vi "RunStimOnRailsThenOnTurns.vi"() -> ()   [LabVIEW 2019]
uses:
  Parameters.ctl
  StimOnRailsThenOnTurns/StimOnRailsThenOnTurnsInputCluster.ctl
  DetectSuppressionDuration/StimOnRailsThenOnTurns.lvclass
  D:/Github_repos/ProjectAPI/LabviewVIs/StimulusObject.lvclass
panel:
  in  "StimOnRailsThenOnTurnsInputCluster":T1={"Constant Intensity (uW/mm^2, negative is blue)"=0.0, "dot radius (mm)"=0.3, "Intensities (uW/mm^2, negative is blue)"=[], "Durations (s)"=[], "Inter trigger interval (s)"=10.0, "Ellipse Ratio Trigger Point"=5.0, "Delays (s)"=[]}
  out "error IO":errorcluster
  in  "SSH password 2":string
  in  "SSH user name 2":string
  in  "Start":bool
  in  "Wait Before Recording (s)":u32
  in  "SSH password":string
  in  "SSH user name":string
  in  "Last Experiment of the Day":bool
  in  "Tags":string
  out "Parameters":T2 {"FW_WormLengthSD" format="%#.6e"}
  # "Faux Worm Drawing"
  # "Tracking"
  # "Temporal Calibration"
  # "Stimulus Generation"
  # "Median Filtering"
  # "Experimental Settings"
  # "Camera and Projector Settings"
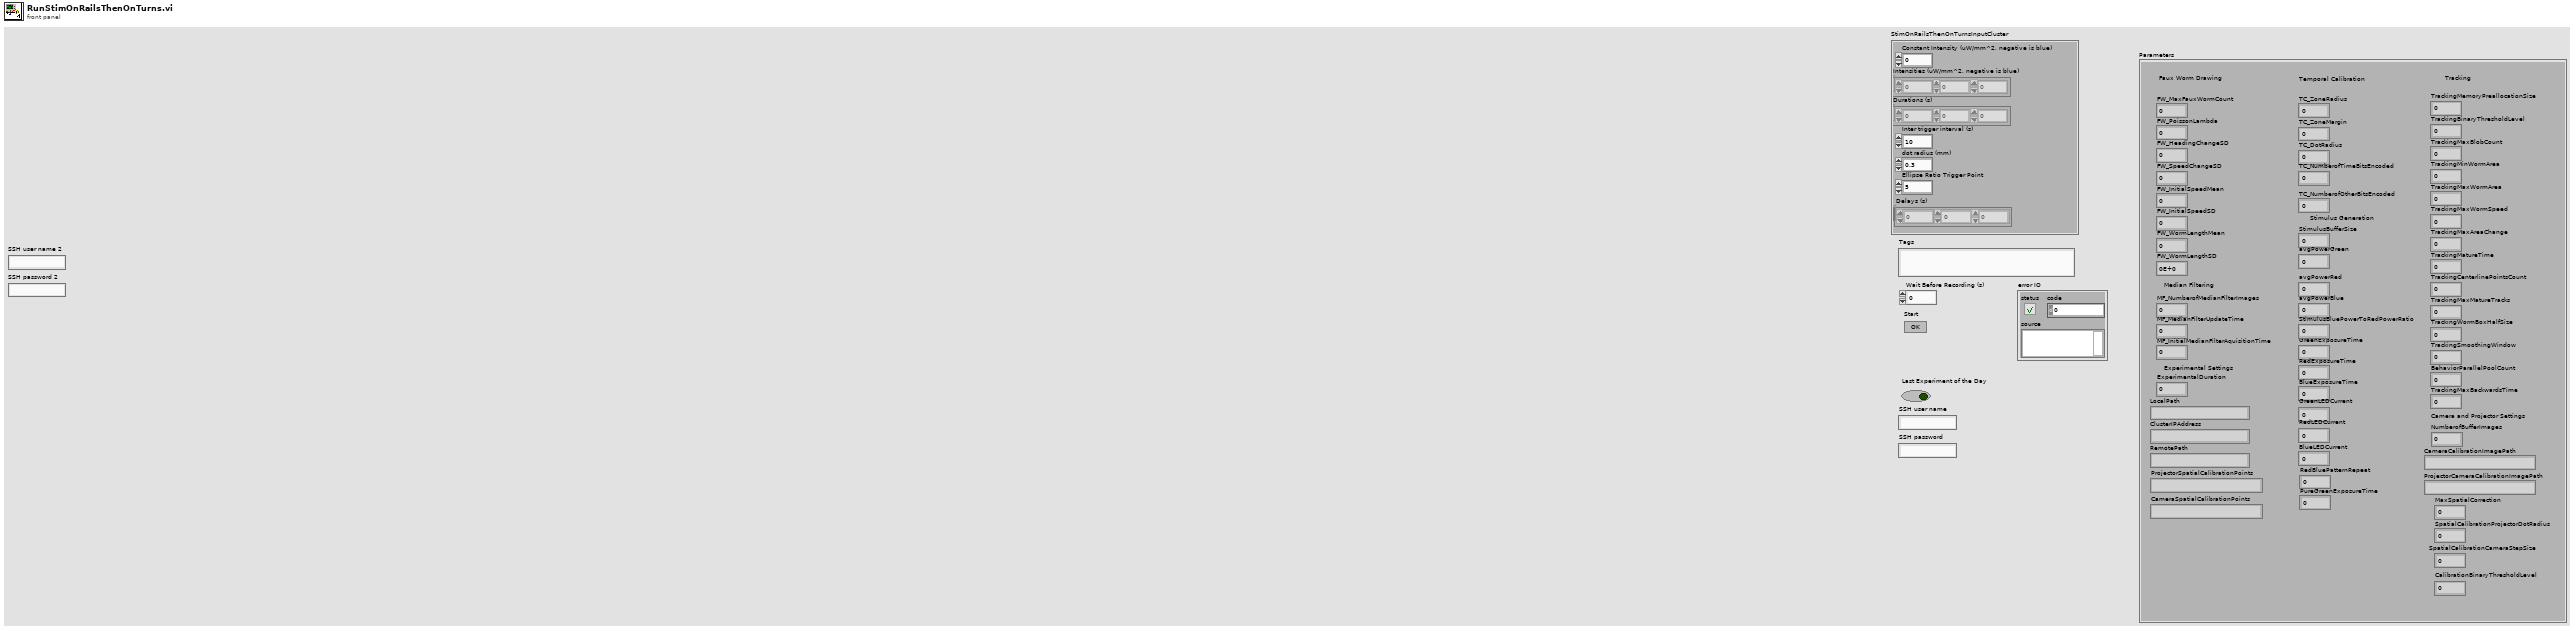
[diagram p1: front panel]
types:
  T1 = typedef "StimOnRailsThenOnTurns.lvclass/StimOnRailsThenOnTurnsInputCluster.ctl" = cluster{"Constant Intensity (uW/mm^2, negative is blue)":sgl, "dot radius (mm)":sgl, "Intensities (uW/mm^2, negative is blue)":sgl[], "Durations (s)":sgl[], "Inter trigger interval (s)":dbl, "Ellipse Ratio Trigger Point":sgl, "Delays (s)":sgl[]}
  T2 = typedef "Parameters.ctl" = cluster{"FW_MaxFauxWormCount":i32, "FW_PoissonLambda":dbl, "FW_HeadingChangeSD":dbl, "FW_SpeedChangeSD":dbl, "FW_InitialSpeedMean":dbl, "FW_InitialSpeedSD":dbl, "FW_WormLengthMean":dbl, "FW_WormLengthSD":dbl, "MF_NumberofMedianFilterImages":i32, "MF_MedianFilterUpdateTime":i32, "MF_InitialMedianFilterAquisitionTime":dbl, "ExperimentalDuration":i32, "TC_ZoneRadius":i32, "TC_ZoneMargin":i32, "TC_DotRadius":dbl, "TC_NumberofTimeBitsEncoded":i32, "TC_NumberofOtherBitsEncoded":i32, "NumberofBufferImages":sgl, "CameraCalibrationImagePath":string, "ProjectorCameraCalibrationImagePath":string, "StimulusBufferSize":i32, "TrackingMemoryPreallocationSize":i32, "TrackingBinaryThresholdLevel":sgl, "TrackingMaxBlobCount":i32, "TrackingMinWormArea":dbl, "TrackingMaxWormArea":dbl, "TrackingMaxWormSpeed":dbl, "TrackingMaxAreaChange":dbl, "TrackingMatureTime":i32, "TrackingCenterlinePointsCount":i32, "TrackingMaxMatureTracks":i32, "TrackingWormBoxHalfSize":i32, "TrackingSmoothingWindow":i32, "BehaviorParallelPoolCount":i32, "LocalPath":string, "GreenExposureTime":i32, "RedExposureTime":i32, "BlueExposureTime":i32, "ClusterIPAddress":string, "RemotePath":string, "GreenLEDCurrent":u8, "RedLEDCurrent":u8, "BlueLEDCurrent":u8, "avgPowerGreen":sgl, "avgPowerRed":sgl, "avgPowerBlue":sgl, "StimulusBluePowerToRedPowerRatio":sgl, "TrackingMaxBackwardsTime":i32, "MaxSpatialCorrection":dbl, "ProjectorSpatialCalibrationPoints":string, "SpatialCalibrationProjectorDotRadius":i32, "SpatialCalibrationCameraStepSize":dbl, "CameraSpatialCalibrationPoints":string, "CalibrationBinaryThresholdLevel":dbl, "RedBluePatternRepeat":i32, "PureGreenExposureTime":i32}
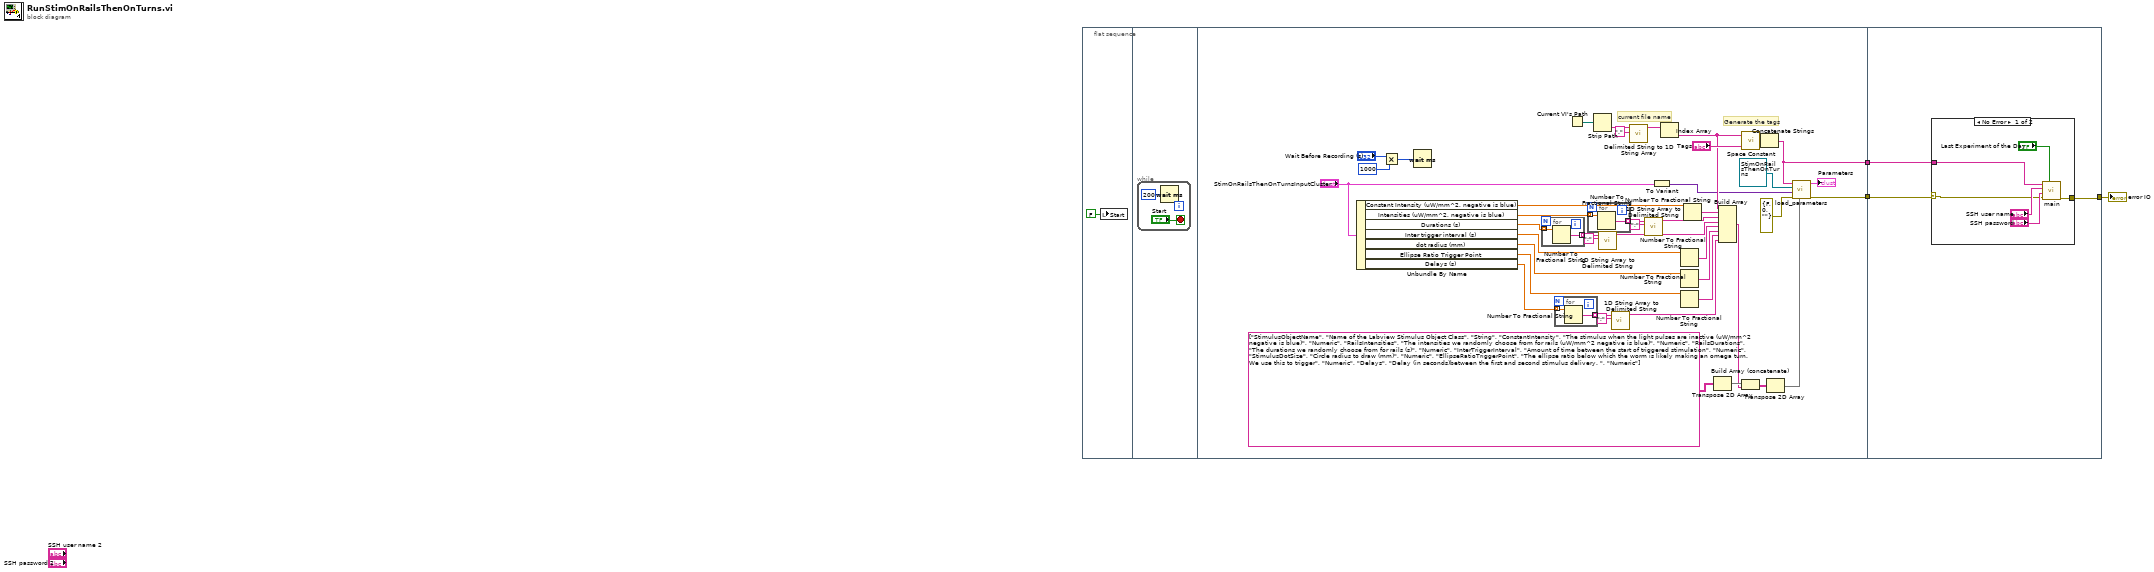
[diagram p0: block diagram]
diagram:
  n1 = flat-sequence {
    tunnel: [w48] -> w3
    tunnel: [w39] -> w2
    tunnel: w2 -> [w56]
    tunnel: w3 -> [w57]
    tunnel: [w55] -> w1
    frame #0 {
      n2 = local write "Start"(FALSE ("Start")) -> ()
    }
    frame #1 {
      n3 = while {
        stop <- "Start" stop-if-true
        n4 = Wait (ms)(milliseconds to wait=u32 200) -> ()  [unwired: 1 out]
      }
    }
    frame #2 {
      # "current file name"
      # "Generate the tags"
      n5 = Unbundle By Name("StimOnRailsThenOnTurnsInputCluster") -> ("Constant Intensity (uW/mm^2, negative is blue)"=w28:sgl, "Intensities (uW/mm^2, negative is blue)"=w27:sgl[], "Durations (s)"=w21:sgl[], "Inter trigger interval (s)"=w18:dbl, "dot radius (mm)"=w19:sgl, "Ellipse Ratio Trigger Point"=w15:sgl, "Delays (s)"=w7:sgl[])
      n6 = Multiply(x="Wait Before Recording (s)", y=u32 1000) -> (x*y=w36:u32)
      n7 = Wait (ms)(milliseconds to wait=w36) -> ()  [unwired: 1 out]
      n8 = for {
        tunnel: w21 -> [w52] mode=indexing
        tunnel: [w51] -> w23 mode=indexing
        n9 = Number To Fractional String(number=w52) -> (F-format string=w51:string)  [unwired: 3 in]
      }
      n10 = for {
        tunnel: w7 -> [w50] mode=indexing
        tunnel: [w49] -> w10 mode=indexing
        n11 = Number To Fractional String(number=w50) -> (F-format string=w49:string)  [unwired: 3 in]
      }
      n12 = Current VI's Path() -> (path=w34:path)
      n13 = for {
        tunnel: w27 -> [w54] mode=indexing
        tunnel: [w53] -> w26 mode=indexing
        n14 = Number To Fractional String(number=w54) -> (F-format string=w53:string)  [unwired: 3 in]
      }
      n15 = Strip Path(path=w34) -> (name=w33:string)  [unwired: 1 out]
      n16 = call <vilib>:"1D String Array to Delimited String.vi"("delimiter"=";", "string array"=w23) -> ("delimited string"=w20:string)  [unwired: 9 in]
      n17 = call <vilib>:"1D String Array to Delimited String.vi"("delimiter"=";", "string array"=w10) -> ("delimited string"=w8:string)  [unwired: 9 in]
      n18 = call <vilib>:"Delimited String to 1D String Array.vi"("delimiter"=".", "delimited string"=w33) -> ("string array"=w31:string[])  [unwired: 9 in]
      n19 = call <vilib>:"1D String Array to Delimited String.vi"("delimiter"=";", "string array"=w26) -> ("delimited string"=w24:string)  [unwired: 9 in]
      n20 = To Variant(anything="StimOnRailsThenOnTurnsInputCluster") -> (Variant=w29:variant)
      n21 = Index Array(array=w31) -> (element=w30:string)  [unwired: 1 in]
      n22 = Number To Fractional String(number=w18) -> (F-format string=w17:string)  [unwired: 3 in]
      n23 = Number To Fractional String(number=w19) -> (F-format string=w16:string)  [unwired: 3 in]
      n24 = Number To Fractional String(number=w15) -> (F-format string=w14:string)  [unwired: 3 in]
      n25 = Number To Fractional String(number=w28) -> (F-format string=w46:string)  [unwired: 3 in]
      n26 = Transpose 2D Array(2D array=string[][] [["StimulusObjectName", "Name of the Labview Stimulus Object Class", "String"], ["ConstantIntensity", "The stimulus when the light pulses are inactive (uW/mm^2 negative is blue)", "Numeric"], ["RailsIntensities", "The intensities we randomly choose from for rails (uW/mm^2 negative is blue)", "Numeric"], ["RailsDurations", "The durations we randomly choose from for rails (s)", "Numeric"], ["InterTriggerInterval", "Amount of time between the start of triggered stimulation", "Numeric"], ["StimulusDotSize", "Circle radius to draw (mm)", "Numeric"], ["EllipseRatioTriggerPoint", "The ellipse ratio below which the worm is likely making an omega turn. We use this to trigger", "Numeric"], ["Delays", "Delay (in seconds)between the first and second stimulus delivery. ", "Numeric"]]) -> (transposed array=w45:string[][])
      n27 = Build Array(w30, w46, w24, w20, w17, w16, w14, w8) -> (w44:string[])
      n28 = Build Array (concatenate)(w45, w44) -> (w43:string[][])
      n29 = call <vilib>:"Space Constant.vi"() -> ("String"=w41:string)
      n30 = Concatenate Strings(w30, w41, "Tags") -> (w39:string)
      n31 = Transpose 2D Array(2D array=w43) -> (transposed array=w40:string[][])
      n32 = call "load_parameters.vi"("additional loaded parameters to write"=w40, "error in (no error)"=errorcluster {"status"=FALSE, "code"=0, "source"=""}, "StimulusObject Parameters"=w29, "StimulusObjectClassInput"=refnum<class "StimOnRailsThenOnTurns.lvclass"> refnum ("StimOnRailsThenOnTurns.lvclass"), "Tags"=w39) -> ("error out"=w48:errorcluster, "Parameters"=→"Parameters":T2)  [unwired: 4 in, 1 out]
    }
    frame #3 {
      n33 = case shown="No Error" w57 {
        selector: w57 -> [w60 w64]
        tunnel: [w59 w64] -> w55
        tunnel: w56 -> [w58 _]
        frame No Error {
          n34 = call "main.vi"("Last Experiment of the Day"="Last Experiment of the Day", "error in"=w60, "SSH password"="SSH password", "SSH user name"="SSH user name", "Tags"=w58) -> ("error out"=w59:errorcluster)  [unwired: 6 in]
        }
        frame Error {
        }
      }
    }
  }
  "error IO" <- w1
